vi "CDK_8xx_900_Project_BuildInfo.vi"(7 "StorageAction":T1, 8 "ErrIn":errorcluster, 10 "BldInfoIn":cluster{"BuildID":string, "DestID":string}[](array[cluster]), 11 "WizardIn":T2) -> (0 "ErrOut":errorcluster, 2 "BldInfoOut":cluster{"BuildID":string, "DestID":string}[](array[cluster]), 3 "WizardOut":T2)   [LabVIEW 2020]
uses:
  <resource>/Framework/Providers/Builds/Installer/CDK_sTypeDef_StorageReadWrite.ctl
  <resource>/Framework/Providers/API/ItemRef.ctl
panel:
  # "Disconnected from typedef"
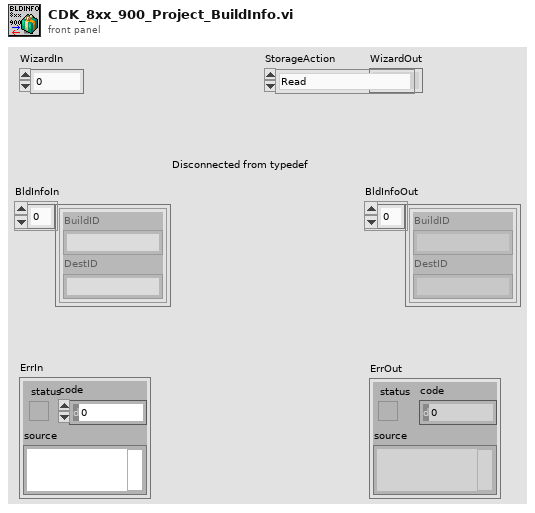
[diagram p1: front panel]
types:
  T1 = typedef "CDK_sTypeDef_StorageReadWrite.ctl" = enum16{"Read", "Write", "Empty", "readPrevious"}
  T2 = typedef "ItemRef.ctl" = u64
  T3 = typedef "CDK_sTypeDef_FileInfo.ctl" = cluster{"FileTag":string, "FileName":string, "Attributes":i16, "RegCOM":bool, "Type":T4, "TypeID":string, "runEXE":bool, "cmdArg":string, "str ref?":bool}
  T4 = typedef "CDK_sTypeDef_BuildTypes.ctl" = enum16{"Invalid", "File", "Folder", "BuildRule", "Library"}
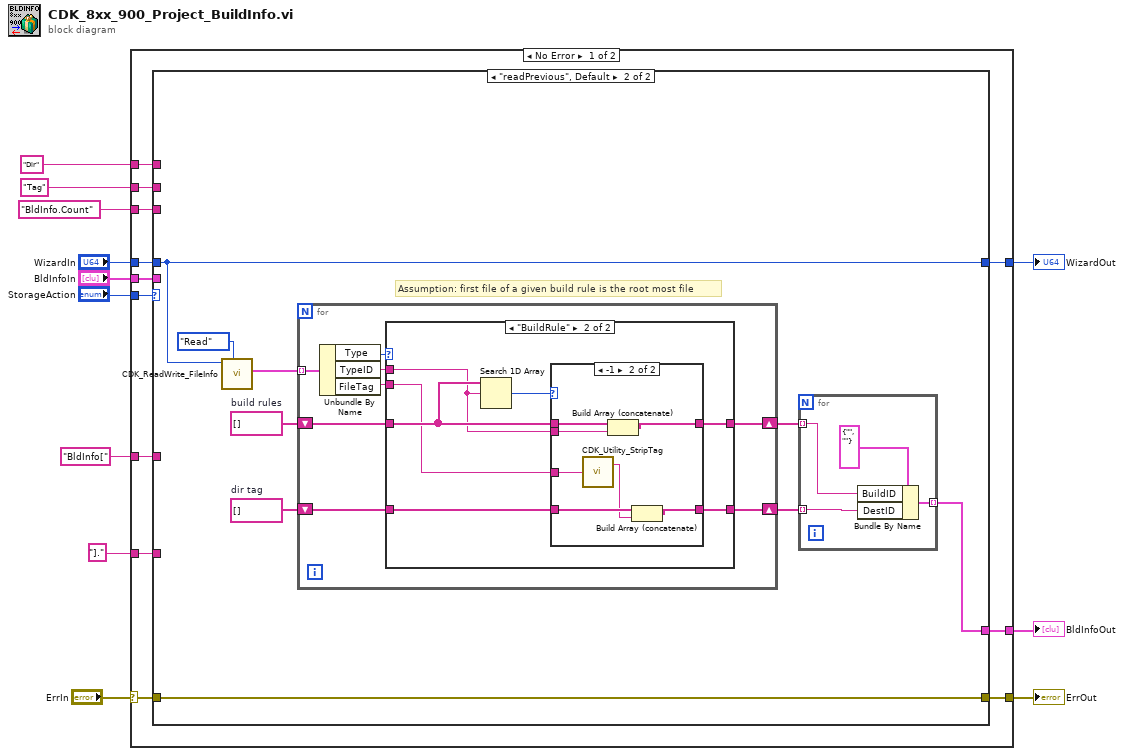
[diagram p0: block diagram]
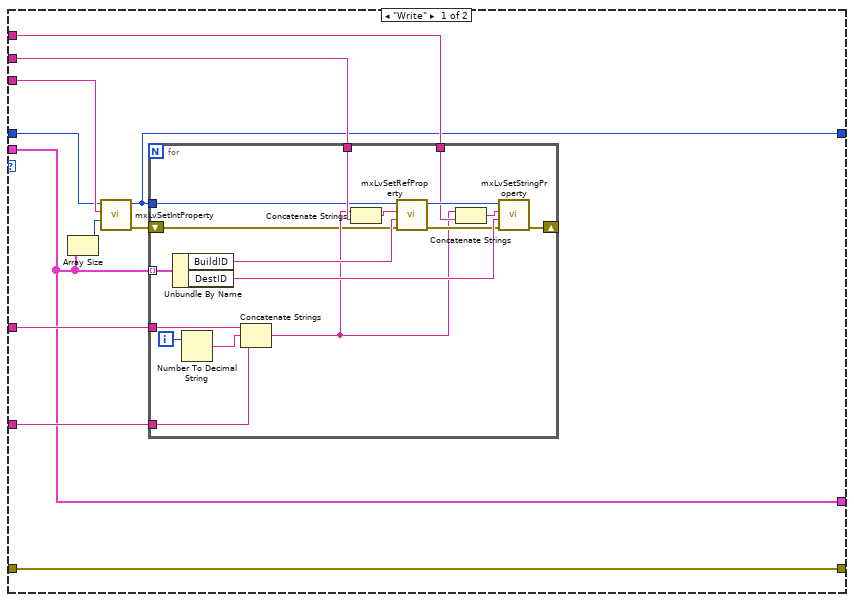
[diagram p2: hidden frame]
diagram:
  n1 = case shown="No Error" "ErrIn" {
    selector: "ErrIn" -> [w21 w94]
    tunnel: [w20 w94] -> w11
    tunnel: "StorageAction" -> [w24 _]
    tunnel: "WizardIn" -> [w23 w93]
    tunnel: "BldInfoIn" -> [w22 w92]
    tunnel: [w19 w93] -> w8
    tunnel: [w18 w92] -> w1
    tunnel: "BldInfo.Count" ("Tag") -> [w17 _]
    tunnel: "Tag" ("Tag") -> [w16 _]
    tunnel: "Dir" ("Tag") -> [w15 _]
    tunnel: "BldInfo[" -> [w14 _]
    tunnel: "]." -> [w13 _]
    frame No Error {
      n2 = case shown="\"readPrevious\", Default" w24 {
        tunnel: w23 -> [w26 w55]
        tunnel: w22 -> [w25 _]
        tunnel: w21 -> [w35 w61]
        tunnel: [w35 w61] -> w20
        tunnel: [w30 w55] -> w19
        tunnel: [w25 w60] -> w18
        tunnel: w17 -> [w33 _]
        tunnel: w16 -> [w32 _]
        tunnel: w15 -> [w31 _]
        tunnel: w14 -> [w28 _]
        tunnel: w13 -> [w27 _]
        frame "Write" {
          n3 = Array Size(array=w25) -> (size(s)=w34:i32)
          n4 = call <resource>:"mxLvSetIntProperty.vi"("Value (0)"=w34, "Tag"=w33, "Item"=w26) -> ("error out"=w29:errorcluster, "Item"=w30:T2)  [unwired: 2 in, 5 out]
          n5 = for {
            tunnel: w25 -> [w52] mode=indexing
            tunnel: w28 -> [w50]
            tunnel: w27 -> [w48]
            tunnel: w30 -> [w37]
            tunnel: w32 -> [w41]
            tunnel: w31 -> [w40]
            shift-right: [w36] -> _
            shift-left: w29 -> [w38]
            i -> [w51]
            n6 = Unbundle By Name(w52) -> ("BuildID"=w43:string, "DestID"=w44:string)
            n7 = Number To Decimal String(number=w51) -> (decimal integer string=w49:string)  [unwired: 1 out]
            n8 = Concatenate Strings(w50, w49, w48) -> (w39:string)
            n9 = Concatenate Strings(w39, w41) -> (w47:string)
            n10 = call <resource>:"mxLvSetRefProperty.vi"("error in"=w38, "Value (\"\")"=w43, "Tag"=w47, "Item"=w37) -> ("error out"=w42:errorcluster, "Item"=w45:T2)  [unwired: 1 in, 5 out]
            n11 = Concatenate Strings(w39, w40) -> (w46:string)
            n12 = call <resource>:"mxLvSetStringProperty.vi"("error in"=w42, "Value (\"\")"=w44, "Tag"=w46, "Item"=w45) -> ("error out"=w36:errorcluster)  [unwired: 1 in, 6 out]
          }
        }
        frame "readPrevious", Default {
          w59 = string[] []  # dir tag
          w58 = string[] []  # build rules
          # "Assumption: first file of a given build rule is the root most file"
          n13 = call <resource>:"CDK_ReadWrite_FileInfo.vi"("StorageAction"=CDK_sTypeDef_StorageReadWrite."Read", "ObjectIn"=w55) -> ("FileInfoOut"=w56:T3[])  [unwired: 2 in, 7 out]
          n14 = for {
            tunnel: w56 -> [w69] mode=indexing
            shift-right: [w62] -> w53
            shift-left: w59 -> [w63]
            shift-right: [w65] -> w54
            shift-left: w58 -> [w67]
            n15 = Unbundle By Name(w69) -> ("Type"=w68:T4, "TypeID"=w66:string, "FileTag"=w64:string)
            n16 = case shown="\"BuildRule\"" w68 {
              tunnel: w67 -> [w71 w78]
              tunnel: w66 -> [_ w76]
              tunnel: [w71 w75] -> w65
              tunnel: w64 -> [_ w74]
              tunnel: w63 -> [w70 w73]
              tunnel: [w70 w72] -> w62
              frame "Invalid", Default {
              }
              frame "BuildRule" {
                n17 = Search 1D Array(1D array=w78, element=w76) -> (index of element=w77:i32)  [unwired: 1 out]
                n18 = case shown="-1" w77 {
                  tunnel: w78 -> [w80 w87]
                  tunnel: w76 -> [_ w86]
                  tunnel: [w80 w85] -> w75
                  tunnel: w74 -> [_ w84]
                  tunnel: w73 -> [w79 w83]
                  tunnel: [w79 w81] -> w72
                  frame Default {
                  }
                  frame -1 {
                    n19 = call <resource>:"CDK_Utility_StripTag.vi"("Path"=w84) -> ("stripped path"=w82:string)  [unwired: 1 in, 1 out]
                    n20 = Build Array (concatenate)(w87, w86) -> (w85:string[])
                    n21 = Build Array (concatenate)(w83, w82) -> (w81:string[])
                  }
                }
              }
            }
          }
          n22 = for {
            tunnel: [w90] -> w60 mode=indexing
            tunnel: w54 -> [w89] mode=indexing
            tunnel: w53 -> [w88] mode=indexing
            n23 = Bundle By Name(cluster=cluster{"BuildID":string, "DestID":string} {"BuildID"="", "DestID"=""} ("BuildInfo"), "BuildID"=w89, "DestID"=w88) -> (w90:cluster{"BuildID":string, "DestID":string})
          }
        }
      }
    }
    frame Error {
    }
  }
  "WizardOut" <- w8
  "ErrOut" <- w11
  "BldInfoOut" <- w1
